vi "Status.get.vi"(8 "error in (no error)":errorcluster, 11 "ComicVine_manager in":refnum<class "ComicVine_manager.lvclass">) -> (0 "error out":errorcluster, 2 "current status":T1, 3 "ComicVine_manager out":refnum<class "ComicVine_manager.lvclass">)   [LabVIEW 2024, in "ComicVine_manager.lvclass"]
uses:
  ComicVine_manager.lvclass
  ComicVine_manager.lvclass/ComicVine_manager.ctl
  status--cluster.ctl
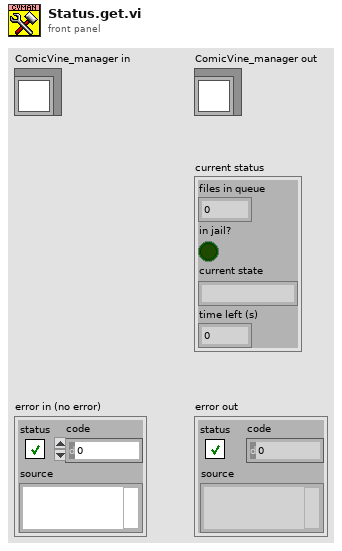
[diagram p1: front panel]
types:
  T1 = typedef "ComicVine_manager.lvclass/status--cluster.ctl" = cluster{"files in queue":i32, "in jail?":bool, "current state":string, "time left (s)":dbl}
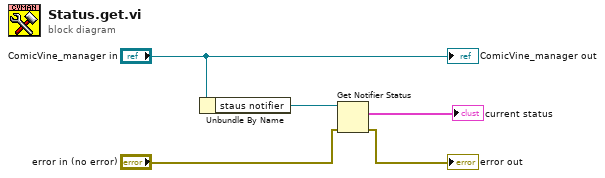
[diagram p0: block diagram]
diagram:
  n1 = Unbundle By Name("ComicVine_manager in") -> ("staus notifier"=w4:refnum<notifier>)
  n2 = Get Notifier Status(notifier=w4, error in (no error)="error in (no error)") -> (current notification=→"current status":T1, error out=→"error out":errorcluster)  [unwired: 3 out]
  "ComicVine_manager out" <- "ComicVine_manager in"
